vi "Configure Correction and Temperature.vi"(8 "error in (no error)":errorcluster, 9 "High Temperature Mode (F: Disable)":bool, 10 "System Error Correction (T: Enable)":bool=TRUE, 11 "VISA resource name":refnum<visa-resource-name>) -> (0 "error out":errorcluster, 3 "VISA resource name out":refnum<visa-resource-name>)   [LabVIEW 2018, in "Agilent ENA Series.lvlib"]
doc: "Configures correction and temperature.\n\nNote:\nThe E5080A does not support the control High Temperature Mode."
uses:
  Agilent ENA Series.lvlib
panel:
  # "Note:\nThe E5080A does not support the control \nHigh Temperature Mode."
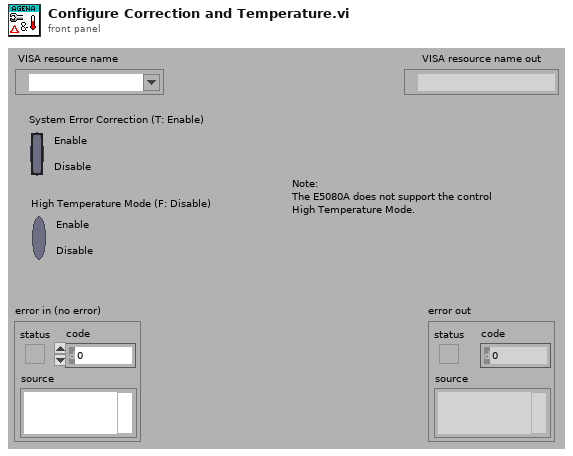
[diagram p1: front panel]
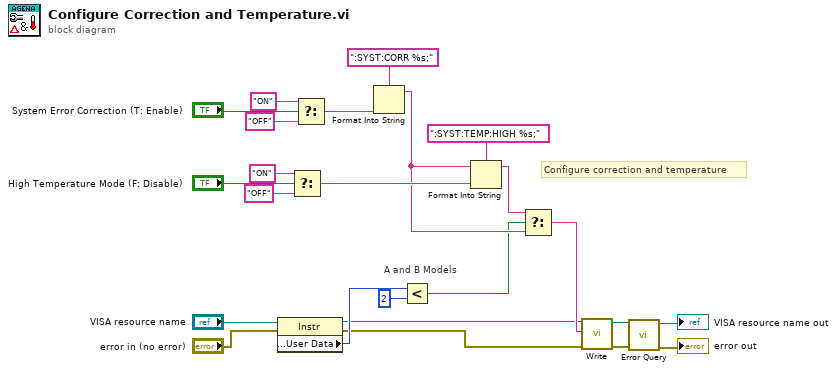
[diagram p0: block diagram]
diagram:
  # "Configure correction and temperature"
  # "A and B Models"
  n1 = property on="Property Node" class="Instr"(reference="VISA resource name", error in="error in (no error)") -> (reference out=w3:refnum<visa-resource-name>, error out=w2:errorcluster, "General Settings:User Data"=w6:u32)
  n2 = Select(t="ON", s="High Temperature Mode (F: Disable)", f="OFF") -> (s? t:f=w11:string)
  n3 = Select(t="ON", s="System Error Correction (T: Enable)", f="OFF") -> (s? t:f=w17:string)
  n4 = Format Into String(format string=":SYST:CORR %s;", w17) -> (resulting string=w9:string)  [unwired: 2 in, 1 out]
  n5 = Less?(x=w6, y=u32 2) -> (x < y?=w1:bool)
  n6 = Format Into String(format string=":SYST:TEMP:HIGH %s;", initial string=w9, w11) -> (resulting string=w10:string)  [unwired: 1 in, 1 out]
  n7 = Select(t=w10, s=w1, f=w9) -> (s? t:f=w4:string)
  n8 = call "Write.vi"("error in (no error)"=w2, "String ()"=w4, "VISA resource name"=w3) -> ("error out"=w15:errorcluster, "VISA resource name out"=w16:refnum<visa-resource-name>)  [unwired: 6 in, 1 out]
  n9 = call "Error Query.vi"("error in (no error)"=w15, "VISA resource name"=w16) -> ("error out"=→"error out":errorcluster, "VISA resource name out"=→"VISA resource name out":refnum<visa-resource-name>)  [unwired: 6 in, 2 out]
